vi "SDK2 multiple cameras.vi"() -> ()   [LabVIEW 2018]
uses:
  Andor SDK/Copy of Andor SDK.lvlib
panel:
  out "Shutdown":u32[](array[numeric])
  out "Initialise":u32[](array[numeric])
  out "Camera Serial numbers available":u32[](array[numeric])
  out "Camera Handles":i32[](array[numeric])
  in  "Shut Down":bool
  out "Current camera":i32
  out "Current Handle":i32
  out "totalCameras":i32
  # "This Example demonstrates how to initialise and \nshutdown multiple cameras in a single application"
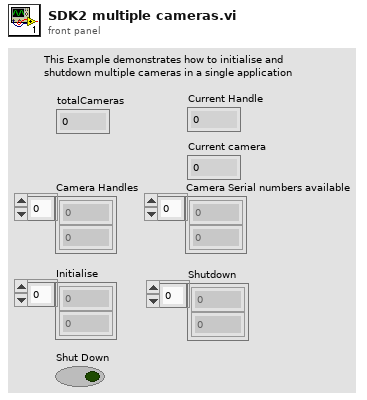
[diagram p1: front panel]
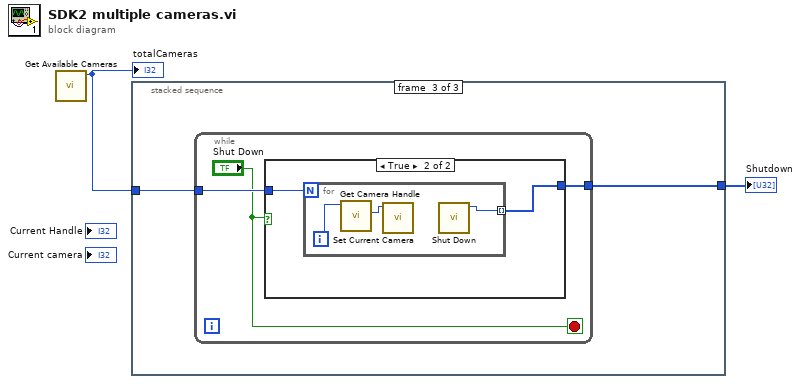
[diagram p0: block diagram]
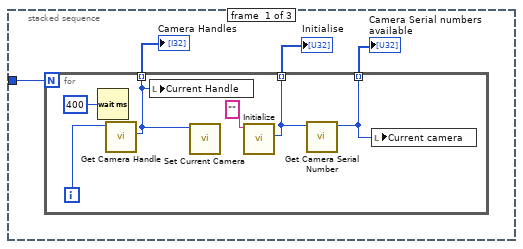
[diagram p2: hidden frame]
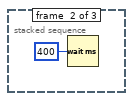
[diagram p3: hidden frame]
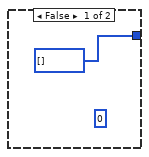
[diagram p4: hidden frame]
diagram:
  n1 = call "Get Available Cameras.vi"() -> ("totalCameras out"=w2:i32)  [unwired: 10 in, 1 out]
  "totalCameras" <- w2
  n2 = stacked-sequence {
    tunnel: w2 -> [w3 _ w14]
    tunnel: [_ _ w15] -> w1
    frame #0 {
      n3 = for {
        N: w3 -> [_]
        tunnel: [w11] -> w6 mode=indexing
        tunnel: [w9] -> w5 mode=indexing
        tunnel: [w7] -> w4 mode=indexing
        i -> [w12]
        n4 = Wait (ms)(milliseconds to wait=u32 400) -> ()  [unwired: 1 out]
        n5 = call "Get Camera Handle.vi"("cameraIndex"=w12) -> ("cameraHandle out"=w11:i32)  [unwired: 9 in, 1 out]
        n6 = local write "Current Handle"(w11) -> ()
        n7 = call "Set Current Camera.vi"("cameraHandle"=w11) -> ()  [unwired: 10 in, 1 out]
        n8 = call "Initialize.vi"("dir"="" ("directory (\"\")")) -> ("function return"=w7:u32)  [unwired: 9 in, 1 out]
        n9 = call "Get Camera Serial Number.vi"("number"=w7) -> ("number out"=w9:i32)  [unwired: 9 in, 1 out]
        n10 = local write "Current camera"(w9) -> ()
      }
      "Camera Handles" <- w6
      "Camera Serial numbers available" <- w5
      "Initialise" <- w4
    }
    frame #1 {
      n11 = Wait (ms)(milliseconds to wait=u32 400) -> ()  [unwired: 1 out]
    }
    frame #2 {
      n12 = while {
        tunnel: [w18] -> w15
        tunnel: w14 -> [w17]
        stop <- "Shut Down" stop-if-true
        n13 = case shown="True" "Shut Down" {
          tunnel: [u32[] [] w21] -> w18
          tunnel: w17 -> [_ w20]
          frame False {
            (unwired) u32 0 ("Close")
          }
          frame True {
            n14 = for {
              N: w20 -> [_]
              tunnel: [w24] -> w21 mode=indexing
              i -> [w23]
              n15 = call "Get Camera Handle.vi"("cameraIndex"=w23) -> ("cameraHandle out"=w22:i32)  [unwired: 9 in, 1 out]
              n16 = call "Set Current Camera.vi"("cameraHandle"=w22) -> ()  [unwired: 10 in, 1 out]
              n17 = call "Shut Down.vi"() -> ("function return"=w24:u32)  [unwired: 11 in]
            }
          }
        }
      }
    }
  }
  "Shutdown" <- w1
